vi "Read And Write.vi"(0 "DAQ":tag[](array[tag]), 3 "File Name":string="DAQ.ini", 5 "error in":errorcluster, 8 "data":string[](array[string])=["Feedback", "Control", "Analog_in"], 10 "Enum":enum16{"Read", "Write"}(ring), 11 "Types of Variables":T4(ring)) -> (7 "DAQmx Analog Input Setting":T1, 14 "DAQmx InPut Setting":T2, 15 "DAQmx OutPut Setting":T3, 16 "DAQ":string[](array[string]), 19 "error out":errorcluster)   [LabVIEW 2015]
uses:
  Galobal variable_TI.vi
  <vilib>/Utility/config.llb/Write Key (Boolean).vi
  <vilib>/Utility/config.llb/NI_LVConfig.lvlib
panel:
  out "key names":string[][](array[string])
  # "Digital Input Configuration"
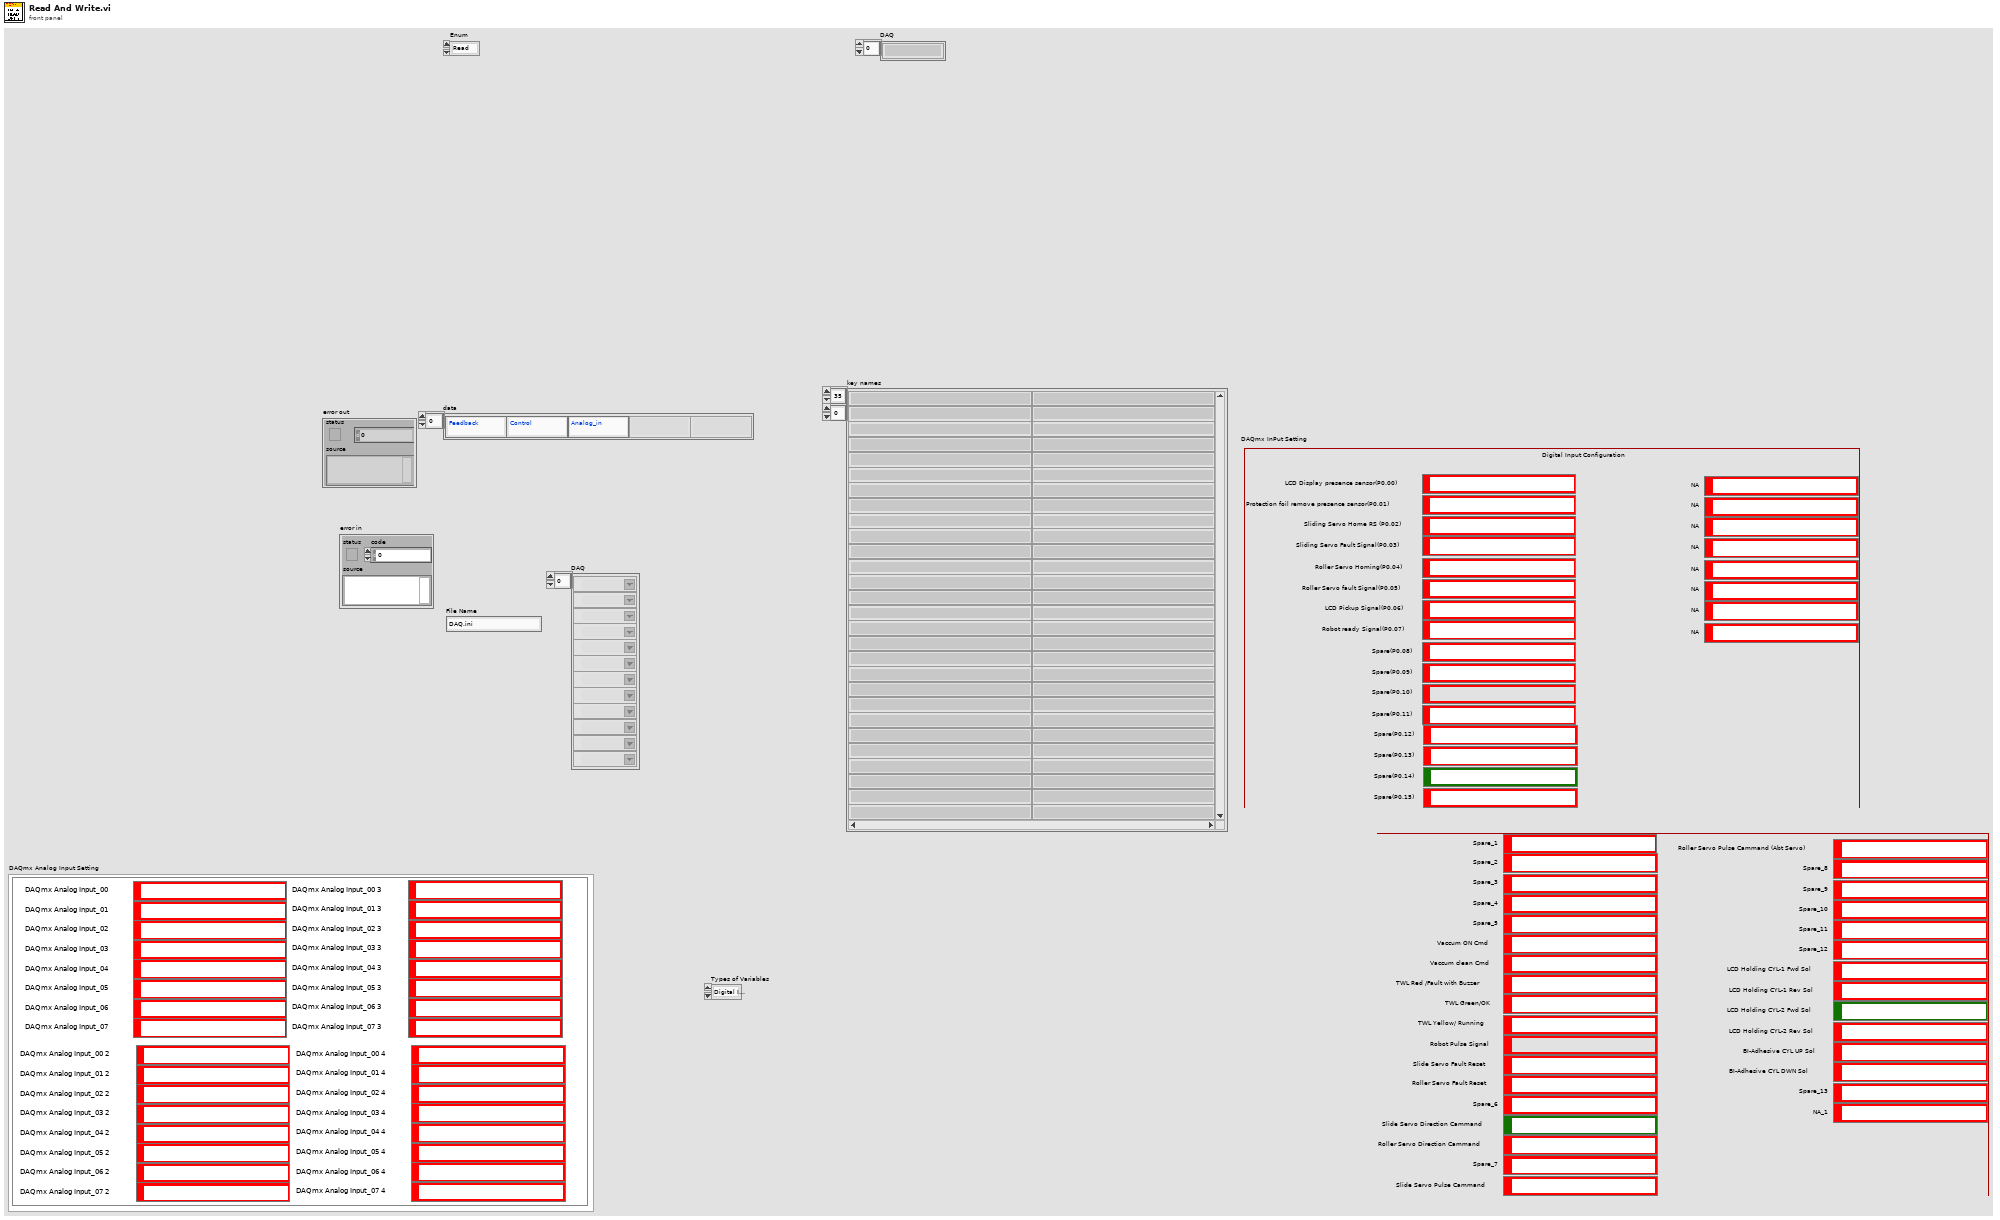
[diagram p1: front panel]
types:
  T1 = cluster{"DAQmx Analog Input_00":tag, "DAQmx Analog Input_01":tag, "DAQmx Analog Input_02":tag, "DAQmx Analog Input_03":tag, "DAQmx Analog Input_04":tag, "DAQmx Analog Input_05":tag, "DAQmx Analog Input_06":tag, "DAQmx Analog Input_07":tag, "DAQmx Analog Input_00 2":tag, "DAQmx Analog Input_01 2":tag, "DAQmx Analog Input_02 2":tag, "DAQmx Analog Input_03 2":tag, "DAQmx Analog Input_04 2":tag, "DAQmx Analog Input_05 2":tag, "DAQmx Analog Input_06 2":tag, "DAQmx Analog Input_07 2":tag, "DAQmx Analog Input_00 3":tag, "DAQmx Analog Input_01 3":tag, "DAQmx Analog Input_02 3":tag, "DAQmx Analog Input_03 3":tag, "DAQmx Analog Input_04 3":tag, "DAQmx Analog Input_05 3":tag, "DAQmx Analog Input_06 3":tag, "DAQmx Analog Input_07 3":tag, "DAQmx Analog Input_00 4":tag, "DAQmx Analog Input_01 4":tag, "DAQmx Analog Input_02 4":tag, "DAQmx Analog Input_03 4":tag, "DAQmx Analog Input_04 4":tag, "DAQmx Analog Input_05 4":tag, "DAQmx Analog Input_06 4":tag, "DAQmx Analog Input_07 4":tag}
  T2 = cluster{"DAQmx InPut_00":tag, "DAQmx InPut_01":tag, "DAQmx InPut_02":tag, "DAQmx InPut_03":tag, "DAQmx InPut_04":tag, "DAQmx InPut_05":tag, "DAQmx InPut_06":tag, "DAQmx InPut_07":tag, "DAQmx InPut_08":tag, "DAQmx InPut_09":tag, "DAQmx InPut_10":tag, "DAQmx InPut_11":tag, "DAQmx InPut_12":tag, "DAQmx InPut_13":tag, "DAQmx InPut_14":tag, "DAQmx InPut_15":tag, "DAQmx InPut_16":tag, "DAQmx InPut_17":tag, "DAQmx InPut_18":tag, "DAQmx InPut_19":tag, "DAQmx InPut_20":tag, "DAQmx InPut_21":tag, "DAQmx InPut_22":tag, "DAQmx InPut_23":tag}
  T3 = cluster{"DAQmx OutPut_00":tag, "DAQmx OutPut_01":tag, "DAQmx OutPut_02":tag, "DAQmx OutPut_03":tag, "DAQmx OutPut_04":tag, "DAQmx OutPut_05":tag, "DAQmx OutPut_06":tag, "DAQmx OutPut_07":tag, "DAQmx OutPut_08":tag, "DAQmx OutPut_09":tag, "DAQmx OutPut_10":tag, "DAQmx OutPut_11":tag, "DAQmx OutPut_12":tag, "DAQmx OutPut_13":tag, "DAQmx OutPut_14":tag, "DAQmx OutPut_15":tag, "DAQmx OutPut_16":tag, "DAQmx OutPut_17":tag, "DAQmx OutPut_18":tag, "DAQmx OutPut_19":tag, "DAQmx OutPut_20":tag, "DAQmx OutPut_21":tag, "DAQmx OutPut_22":tag, "DAQmx OutPut_23":tag, "DAQmx OutPut_12 2":tag, "DAQmx OutPut_13 2":tag, "DAQmx OutPut_14 2":tag, "DAQmx OutPut_15 2":tag, "DAQmx OutPut_16 2":tag, "DAQmx OutPut_17 2":tag, "DAQmx OutPut_18 2":tag, "DAQmx OutPut_19 2":tag}
  T4 = enum16{"Digital Input", "Digital Output", "Analog Input", "Servo Input"}
  T5 = typedef "NI_LVConfig.lvlib/Config Data RefNum.ctl" = refnum<k1>
  T6 = cluster{"key names[0]":string, "key names[1]":string, "key names[2]":string, "key names[3]":string, "key names[4]":string, "key names[5]":string, "key names[6]":string, "key names[7]":string, "key names[8]":string, "key names[9]":string, "key names[10]":string, "key names[11]":string, "key names[12]":string, "key names[13]":string, "key names[14]":string, "key names[15]":string, "key names[16]":string, "key names[17]":string, "key names[18]":string, "key names[19]":string, "key names[20]":string, "key names[21]":string, "key names[22]":string, "key names[23]":string}
  T7 = cluster{"key names[0]":string, "key names[1]":string, "key names[2]":string, "key names[3]":string, "key names[4]":string, "key names[5]":string, "key names[6]":string, "key names[7]":string, "key names[8]":string, "key names[9]":string, "key names[10]":string, "key names[11]":string, "key names[12]":string, "key names[13]":string, "key names[14]":string, "key names[15]":string, "key names[16]":string, "key names[17]":string, "key names[18]":string, "key names[19]":string, "key names[20]":string, "key names[21]":string, "key names[22]":string, "key names[23]":string, "key names[24]":string, "key names[25]":string, "key names[26]":string, "key names[27]":string, "key names[28]":string, "key names[29]":string, "key names[30]":string, "key names[31]":string}
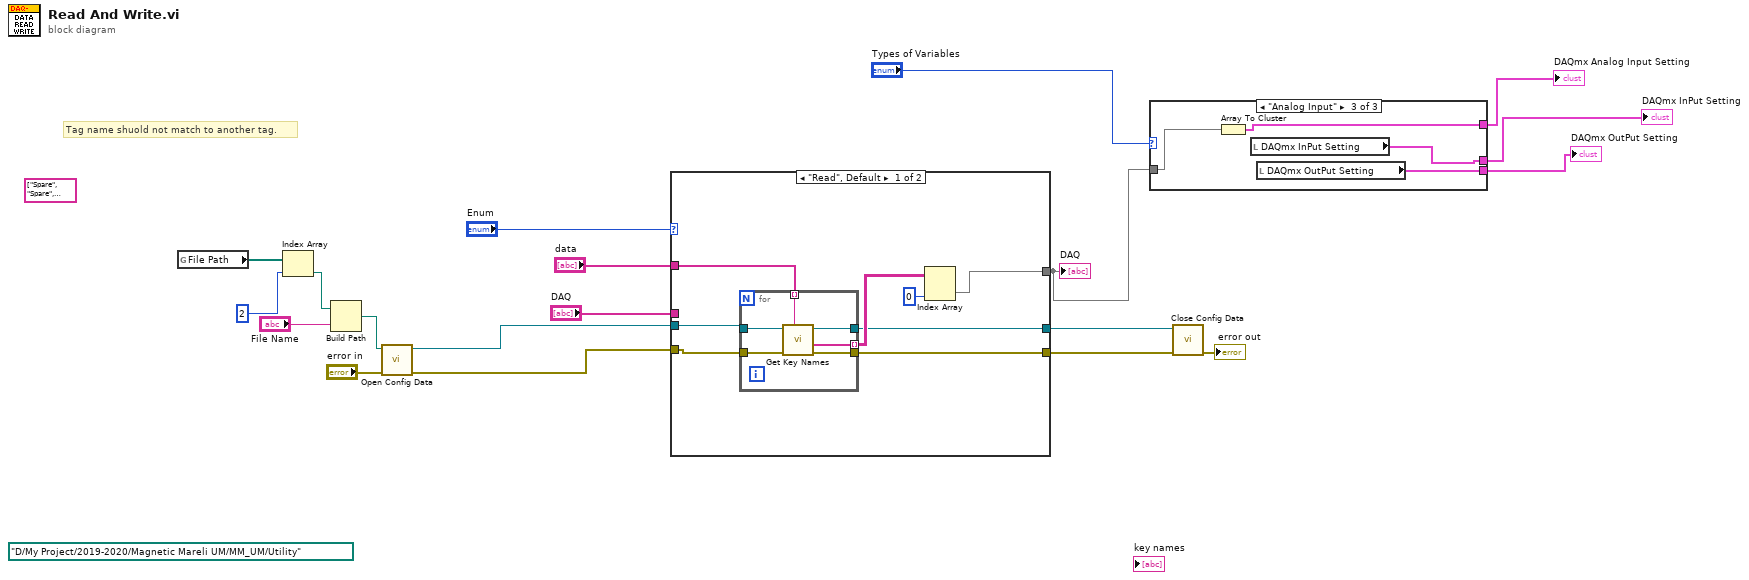
[diagram p0: block diagram]
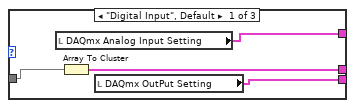
[diagram p2: hidden frame]
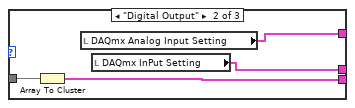
[diagram p3: hidden frame]
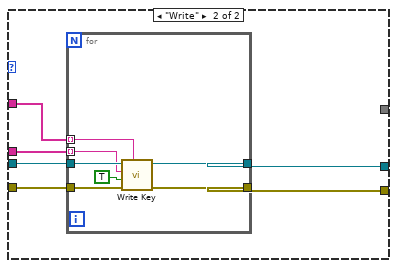
[diagram p4: hidden frame]
diagram:
  (unwired) string[] ["Spare", "Spare", "Spare", "Spare", "Spare", "Vaccum ON Cmd", "Vaccum clean Cmd", "TWL Red /Fault with Buzzer", "TWL Green/OK", "TWL Yellow/ Running", "Robot Pulse Signal", "Slide Servo Fault Reset ", "Roller Servo Fault Reset", "Spare", "Slide Servo Direction Cammand", "Roller Servo Direction Cammand", "Spare", "Slide Servo Pulse Cammand", "Roller Servo Pulse Cammand (Abt Servo)", "Spare", "Spare", "Spare", "Spare", "Spare", "LCD Holding CYL-1 Fwd Sol", "LCD Holding CYL-1 Rev Sol", "LCD Holding CYL-2 Fwd Sol", "LCD Holding CYL-2 Rev Sol", "BI-Adhesive CYL UP Sol", "BI-Adhesive CYL DWN Sol  ", "Spare", "NA", "NA", "NA", "NA", "NA"] ("subarray")
  (unwired) path "D:/My Project/2019-2020/Magnetic Mareli UM/MM_UM/Utility" ("base path")
  # "Tag name shuold not match to another tag."
  n1 = global read "Galobal variable_TI.vi" "File Path"() -> (w12:path[])
  n2 = Index Array(array=w12, index=2) -> (element=w10:path)
  n3 = Build Path(base path=w10, name or relative path="File Name") -> (appended path=w17:path)
  n4 = call <vilib>:"Open Config Data.vi"("error in (no error)"="error in", "configuration file path"=w17) -> ("error out"=w8:errorcluster, "refnum"=w9:T5)  [unwired: 7 in, 1 out]
  n5 = case shown="\"Read\", Default" "Enum" {
    tunnel: [w21 w39] -> w16
    tunnel: [w20 w38] -> w15
    tunnel: "DAQ" -> [_ w37]
    tunnel: w9 -> [w27 w36]
    tunnel: w8 -> [w26 w35]
    tunnel: "data" -> [w25 w34]
    tunnel: [w22 _] -> w4
    frame "Read", Default {
      n6 = for {
        tunnel: w27 -> [w33]
        tunnel: w26 -> [w32]
        tunnel: [w31] -> w24 mode=indexing
        tunnel: w25 -> [w30] mode=indexing
        tunnel: [w29] -> w21
        tunnel: [w28] -> w20
        n7 = call <vilib>:"Get Key Names.vi"("section"=w30, "error in (no error)"=w32, "refnum"=w33) -> ("error out"=w28:errorcluster, "key names"=w31:string[], "refnum out"=w29:T5)  [unwired: 5 in, 1 out]
      }
      n8 = Index Array(array=w24, index (col)=0 ("disabled index (col)")) -> (element=w22:string[])  [unwired: 1 in]
    }
    frame "Write" {
      n9 = for {
        tunnel: w34 -> [w44] mode=indexing
        tunnel: w36 -> [w46]
        tunnel: w35 -> [w45]
        tunnel: w37 -> [w43] mode=indexing
        tunnel: [w42] -> w39
        tunnel: [w41] -> w38
        n10 = call-poly <vilib>:"Write Key.vi"("section"=w44, "error in (no error)"=w45, "value"=TRUE, "key"=w43, "refnum"=w46) -> ("error out"=w41:errorcluster, "refnum out"=w42:T5)  [unwired: 4 in, 1 out]
      }
    }
  }
  "DAQ" <- w4
  n11 = case shown="\"Analog Input\"" "Types of Variables" {
    tunnel: w4 -> [w50 w54 w58]
    tunnel: [w49 w52 w55] -> w3
    tunnel: [w47 w53 w56] -> w2
    tunnel: [w48 w51 w57] -> w1
    frame "Digital Input", Default {
      n12 = local read "DAQmx Analog Input Setting"() -> (w48:T1)
      n13 = Array To Cluster(array=w50) -> (cluster=w49:T6)
      n14 = local read "DAQmx OutPut Setting"() -> (w47:T3)
    }
    frame "Digital Output" {
      n15 = Array To Cluster(array=w54) -> (cluster=w53:T7)
      n16 = local read "DAQmx Analog Input Setting"() -> (w51:T1)
      n17 = local read "DAQmx InPut Setting"() -> (w52:T2)
    }
    frame "Analog Input" {
      n18 = Array To Cluster(array=w58) -> (cluster=w57:T7)
      n19 = local read "DAQmx InPut Setting"() -> (w55:T2)
      n20 = local read "DAQmx OutPut Setting"() -> (w56:T3)
    }
  }
  "DAQmx OutPut Setting" <- w2
  "DAQmx Analog Input Setting" <- w1
  "DAQmx InPut Setting" <- w3
  n21 = call <vilib>:"Close Config Data.vi"("error in (no error)"=w15, "refnum"=w16) -> ("error out"=→"error out":errorcluster)  [unwired: 8 in, 1 out]
